vi "Model Initial Values - Add Model RTM.vi"(8 "error in (no error)":errorcluster, 11 "Node Ptr":u64 format="%.0x") -> (0 "error out":errorcluster)   [LabVIEW 2011, in "Model Initial Values Custom Device.lvlib"]
uses:
  Model Initial Values Custom Device.lvlib
  Model Initial Values - Global.vi
  <vilib>/NI Veristand/Custom Device API/Set Item Property (String Array).vi
  <vilib>/NI Veristand/Custom Device API/Set Item Property (Double Array).vi
  <vilib>/NI Veristand/Custom Device API/Set Item Property (String).vi
  <vilib>/NI Veristand/Custom Device API/Set Item Property (I32).vi
  <vilib>/NI Veristand/Custom Device Tools/Custom Device Utility Library/Custom Device Utility Library.lvlib
  <vilib>/NI Veristand/Custom Device API/Custom Device API.lvlib
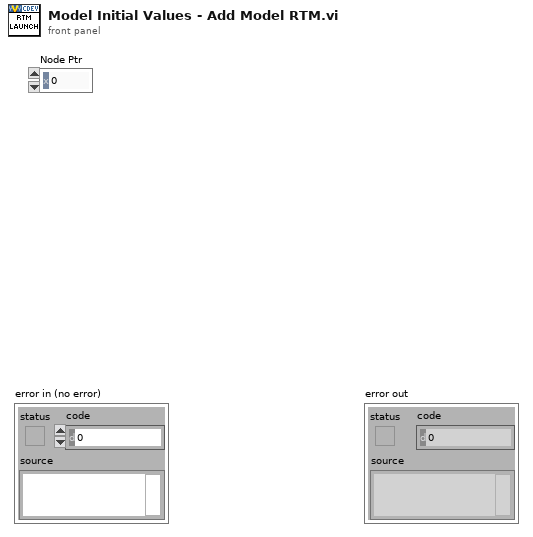
[diagram p1: front panel]
types:
  T1 = typedef "Custom Device API.lvlib/Custom Device Item Ref.ctl" = u64
  T2 = cluster{"Name":string, "Is Channel":bool, "GUID":string}
  T3 = cluster{"DLLSize":i32, "Timestamp":dbl, "MD5":string}
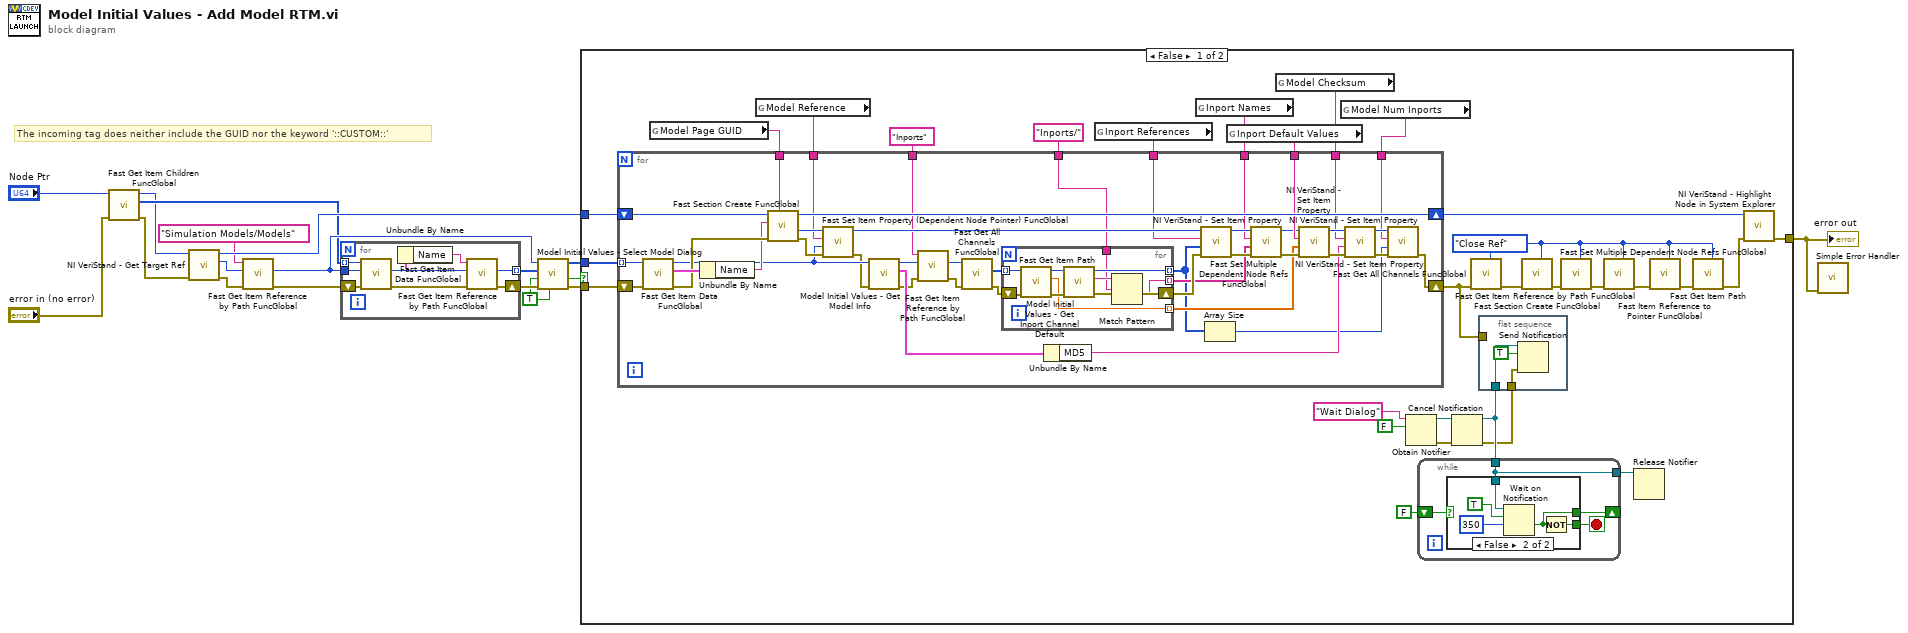
[diagram p0: block diagram]
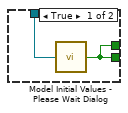
[diagram p2: hidden frame]
diagram:
  w9 = TRUE ("Multi-Selection?")
  # "The incoming tag does neither include the GUID nor the keyword '::CUSTOM::'"
  n1 = call "Fast Get Item Children FuncGlobal.vi"("error in (no error)"="error in (no error)", "Item Ref in"="Node Ptr") -> ("error out"=w7:errorcluster, "Child Refs"=w6:T1[], "Item Ref out"=w5:T1)  [unwired: 6 in, 1 out]
  n2 = call <vilib>:"NI VeriStand - Get Target Ref.vi"("error in"=w7, "Item Ref in"=w5) -> ("error out"=w12:errorcluster, "Target Ref"=w14:T1, "Item Ref out"=w15:T1)  [unwired: 6 in, 1 out]
  n3 = call "Fast Get Item Reference by Path FuncGlobal.vi"("error in (no error)"=w12, "Root Ref"=w14, "Item Path in"="Simulation Models/Models" ("Relative Item Path")) -> ("error out"=w10:errorcluster, "Item Ref"=w11:T1)  [unwired: 5 in, 2 out]
  n4 = for {
    tunnel: w11 -> [w26]
    shift-right: [w25] -> w18
    shift-left: w10 -> [w22]
    tunnel: [w24] -> w17 mode=indexing
    tunnel: w6 -> [w19] mode=indexing
    n5 = call "Fast Get Item Data FuncGlobal.vi"("error in (no error)"=w22, "Item Ref in"=w19) -> ("error out"=w21:errorcluster, "Item Info"=w20:T2)  [unwired: 6 in, 2 out]
    n6 = Unbundle By Name(w20) -> ("Name"=w23:string)
    n7 = call "Fast Get Item Reference by Path FuncGlobal.vi"("error in (no error)"=w21, "Root Ref"=w26, "Item Path in"=w23) -> ("error out"=w25:errorcluster, "Item Ref"=w24:T1)  [unwired: 5 in, 2 out]
  }
  n8 = call "Model Initial Values - Select Model Dialog.vi"("Multi-Selection?"=w9, "error in (no error)"=w18, "Allow Section Selection (F)"=w9, "Initial Selection"=w17, "Root Item Ref"=w11) -> ("error out"=w2:errorcluster, "Canceled"=w1:bool, "Selected Channel Refs"=w16:T1[])  [unwired: 4 in]
  n9 = case shown="False" w1 {
    tunnel: w16 -> [w56 _]
    tunnel: w15 -> [w55 _]
    tunnel: [w52 w124] -> w3
    tunnel: w2 -> [w45 w124]
    frame False {
      w27 = enum16{"Open or Add", "Close Ref"}."Close Ref" ("Action")
      n10 = global read "Model Initial Values - Global.vi" "Model Page GUID"() -> (w42:string)
      n11 = global read "Model Initial Values - Global.vi" "Model Reference"() -> (w43:string)
      n12 = global read "Model Initial Values - Global.vi" "Inport References"() -> (w41:string)
      n13 = global read "Model Initial Values - Global.vi" "Inport Names"() -> (w39:string)
      n14 = global read "Model Initial Values - Global.vi" "Inport Default Values"() -> (w38:string)
      n15 = global read "Model Initial Values - Global.vi" "Model Checksum"() -> (w37:string)
      n16 = global read "Model Initial Values - Global.vi" "Model Num Inports"() -> (w36:string)
      n17 = for {
        tunnel: w56 -> [w111] mode=indexing
        shift-right: [w75] -> w46
        shift-left: w45 -> [w113]
        shift-right: [w107] -> w54
        shift-left: w55 -> [w108]
        tunnel: "Inports" ("Item Path in") -> [w100]
        tunnel: w43 -> [w99]
        tunnel: w42 -> [w98]
        tunnel: w41 -> [w97]
        tunnel: w39 -> [w94]
        tunnel: w38 -> [w91]
        tunnel: w37 -> [w85]
        tunnel: w36 -> [w74]
        tunnel: "Inports/" ("regular expression") -> [w71]
        n18 = call "Fast Get Item Data FuncGlobal.vi"("error in (no error)"=w113, "Item Ref in"=w111) -> ("error out"=w110:errorcluster, "Item Info"=w112:T2, "Item Ref out"=w81:T1)  [unwired: 6 in, 1 out]
        n19 = Unbundle By Name(w112) -> ("Name"=w109:string)
        n20 = call "Fast Section Create FuncGlobal.vi"("GUID (Default Section)"=w98, "error in (no error)"=w110, "Section Name"=w109, "Parent Ref in"=w108) -> ("error out"=w106:errorcluster, "Section Ptr"=w105:T1, "Parent Ref out"=w107:T1)  [unwired: 4 in, 1 out]
        n21 = call "Fast Set Item Property (Dependent Node Pointer) FuncGlobal.vi"("error in (no error)"=w106, "Dependent Node Ref"=w81, "Property Name"=w99, "Item Ref in"=w105) -> ("error out"=w79:errorcluster, "Item Ref out"=w104:T1)  [unwired: 5 in, 1 out]
        n22 = call "Model Initial Values - Get Model Info.vi"("error in (no error)"=w79, "ID in"=w81) -> ("error out"=w80:errorcluster, "output cluster"=w88:T3, "ID out"=w78:T1)  [unwired: 7 in]
        n23 = call "Fast Get Item Reference by Path FuncGlobal.vi"("error in (no error)"=w80, "Root Ref"=w78, "Item Path in"=w100) -> ("error out"=w83:errorcluster, "Item Ref"=w82:T1)  [unwired: 5 in, 2 out]
        n24 = call "Fast Get All Channels FuncGlobal.vi"("error in"=w83, "Section Ref in"=w82) -> ("error out"=w101:errorcluster, "Channel Refs"=w103:T1[])  [unwired: 6 in, 2 out]
        n25 = for {
          tunnel: w103 -> [w123] mode=indexing
          shift-right: [w118] -> w102
          shift-left: w101 -> [w122]
          tunnel: [w119] -> w90 mode=indexing
          tunnel: [w115] -> w93 mode=indexing
          tunnel: [w117] -> w73 mode=indexing
          tunnel: w71 -> [w114]
          n26 = call "Model Initial Values - Get Inport Channel Default.vi"("error in"=w122, "Item Ref in"=w123) -> ("error out"=w120:errorcluster, "Default Value"=w119:dbl, "Item Ref out"=w121:T1)  [unwired: 6 in]
          n27 = call "Fast Get Item Path.vi"("error in (no error)"=w120, "Item Ref in"=w121) -> ("error out"=w118:errorcluster, "Path"=w116:string, "Item Ref out"=w117:T1)  [unwired: 6 in, 1 out]
          n28 = Match Pattern(string=w116, regular expression=w114) -> (after substring=w115:string)  [unwired: 1 in, 3 out]
        }
        n29 = Unbundle By Name(w88) -> ("MD5"=w84:string)
        n30 = call "Fast Set Multiple Dependent Node Refs FuncGlobal.vi"("error in (no error)"=w102, "Dependent Node Refs"=w73, "Base Property Name"=w97, "Item Ref in"=w104) -> ("error out"=w96:errorcluster, "Item Ref out"=w95:T1)  [unwired: 6 in]
        n31 = Array Size(array=w73) -> (size(s)=w72:i32)
        n32 = call-poly <vilib>:"NI VeriStand - Set Item Property.vi"("error in (no error)"=w96, "Value"=w93, "Property Name"=w94, "Item Ref in"=w95) -> ("error out"=w92:errorcluster, "Item Ref out"=w89:T1)  [unwired: 5 in, 1 out]
        n33 = call-poly <vilib>:"NI VeriStand - Set Item Property.vi"("error in (no error)"=w92, "Value"=w90, "Property Name"=w91, "Item Ref in"=w89) -> ("error out"=w87:errorcluster, "Item Ref out"=w86:T1)  [unwired: 5 in, 1 out]
        n34 = call-poly <vilib>:"NI VeriStand - Set Item Property.vi"("error in (no error)"=w87, "Value"=w84, "Property Name"=w85, "Item Ref in"=w86) -> ("error out"=w77:errorcluster, "Item Ref out"=w76:T1)  [unwired: 5 in, 1 out]
        n35 = call-poly <vilib>:"NI VeriStand - Set Item Property.vi"("error in (no error)"=w77, "Value"=w72, "Property Name"=w74, "Item Ref in"=w76) -> ("error out"=w75:errorcluster)  [unwired: 5 in, 2 out]
      }
      n36 = Obtain Notifier(name (unnamed)="Wait Dialog", notification data type=FALSE) -> (notifier out=w47:refnum<notifier>, error out=w32:errorcluster)  [unwired: 2 in, 1 out]
      n37 = Cancel Notification(0:w47, 3:w32) -> (8:w33:refnum<notifier>, 11:w31:errorcluster)  [unwired: 1 out]
      n38 = while {
        tunnel: w33 -> [w60]
        shift-right: [w61] -> _
        shift-left: FALSE -> [w62]
        tunnel: [w60] -> w34
        stop <- w63 stop-if-true
        n39 = case shown="False" w62 {
          tunnel: [w64 w68] -> w63
          tunnel: w60 -> [w65 w70]
          tunnel: [w64 w66] -> w61
          frame True {
            n40 = call "Model Initial Values - Please Wait Dialog.vi"("notifier out"=w65) -> ("Boolean"=w64:bool)
          }
          frame False {
            n41 = Wait on Notification(notifier=w70, ignore previous (F)=TRUE, timeout in ms (-1)=350) -> (timed out?=w66:bool)  [unwired: 1 in, 3 out]
            n42 = Not(x=w66) -> (.not. x?=w68:bool)
          }
        }
      }
      n43 = call "Fast Get All Channels FuncGlobal.vi"("Action"=w27, "error in"=w46) -> ("error out"=w53:errorcluster)  [unwired: 6 in, 3 out]
      n44 = flat-sequence {
        tunnel: w33 -> [w59]
        tunnel: w31 -> [w58]
        tunnel: w46 -> [_]
        frame #0 {
          n45 = Send Notification(notification=TRUE, notifier=w59, error in (no error)=w58) -> ()  [unwired: 2 out]
        }
      }
      n46 = call "Fast Section Create FuncGlobal.vi"("Action"=w27, "error in (no error)"=w53) -> ("error out"=w51:errorcluster)  [unwired: 6 in, 3 out]
      n47 = call "Fast Set Multiple Dependent Node Refs FuncGlobal.vi"("Action"=w27, "error in (no error)"=w51) -> ("error out"=w50:errorcluster)  [unwired: 8 in, 1 out]
      n48 = call "Fast Get Item Reference by Path FuncGlobal.vi"("Action"=w27, "error in (no error)"=w50) -> ("error out"=w40:errorcluster)  [unwired: 6 in, 3 out]
      n49 = Release Notifier(notifier=w34) -> ()  [unwired: 2 in, 3 out]
      n50 = call "Fast Item Reference to Pointer FuncGlobal.vi"("Action"=w27, "error in (no error)"=w40) -> ("error out"=w29:errorcluster)  [unwired: 6 in, 3 out]
      n51 = call "Fast Get Item Path.vi"("Action"=w27, "error in (no error)"=w29) -> ("error out"=w28:errorcluster)  [unwired: 6 in, 3 out]
      n52 = call <vilib>:"NI VeriStand - Highlight Node in System Explorer.vi"("error in (no error)"=w28, "Item Ref in"=w54) -> ("error out"=w52:errorcluster)  [unwired: 8 in, 1 out]
    }
    frame True {
    }
  }
  "error out" <- w3
  n53 = call <vilib>:"Simple Error Handler.vi"("error in (no error)"=w3) -> ()  [unwired: 4 in, 5 out]
